vi "Read Trigger.lvclass.vi"(8 "error in (no error)":errorcluster, 11 "Sync Box in":refnum<class "Sync Box.lvclass">) -> (0 "error out":errorcluster, 2 "Trigger.lvclass":refnum<class "Trigger.lvclass">, 3 "Sync Box out":refnum<class "Sync Box.lvclass">)   [LabVIEW 2012, in "Sync Box.lvclass"]
uses:
  Sync Box.lvclass
  Trigger/Trigger.lvclass
  Sync Box.lvclass/Sync Box.ctl
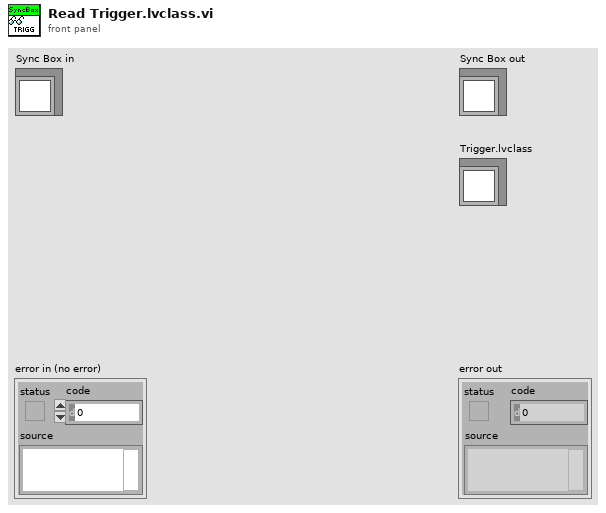
[diagram p1: front panel]
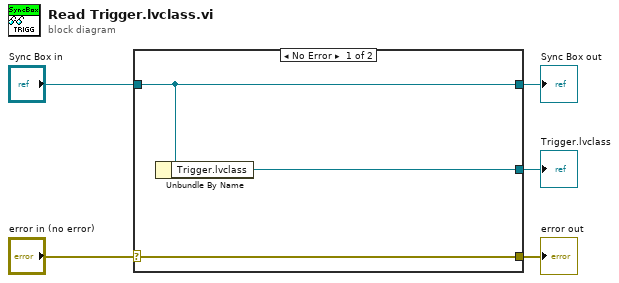
[diagram p0: block diagram]
diagram:
  n1 = case shown="No Error" "error in (no error)" {
    selector: "error in (no error)" -> [w8 w9]
    tunnel: [w8 w9] -> w4
    tunnel: [w7 w10] -> w2
    tunnel: "Sync Box in" -> [w7 w10]
    tunnel: [w6 _] -> w1
    frame No Error {
      n2 = Unbundle By Name(w7) -> ("Trigger.lvclass"=w6:refnum<class "Trigger.lvclass">)
    }
    frame Error {
    }
  }
  "error out" <- w4
  "Sync Box out" <- w2
  "Trigger.lvclass" <- w1
